vi "ConcatenateOntoShortcutMenu.vi"(8 "error in":errorcluster, 9 "menu ref in":refnum<k9>, 11 "Scope in":refnum<class "Scope Instrument.lvclass">) -> (0 "error out":errorcluster, 1 "menu ref out":refnum<k9>, 3 "Scope out":refnum<class "Scope Instrument.lvclass">)   [LabVIEW 2025, in "Scope.lvlib" / "Scope Instrument.lvclass"]
doc: "Allows children to insert menu items without overriding ShortcutMenu.vi entirely. By default, called after Add/Remove.Copyright 2017 National Instruments Corporation\n\nLicensed under the Apache License, Version 2.0 (the \"License\"); you may not use this file except in compliance with the License. You may obtain a copy of the License at http://www.apache.org/licenses/LICENSE-2.0\nUnless required by applicable law or agreed to in writing, software distributed under the License is distributed on an \"AS IS\" BASIS, WITHOUT WARRANTIES OR CONDITIONS OF ANY KIND, either express or implied. See the License for the specific language governing permissions and limitations under the License."
uses:
  Scope Instrument.lvclass
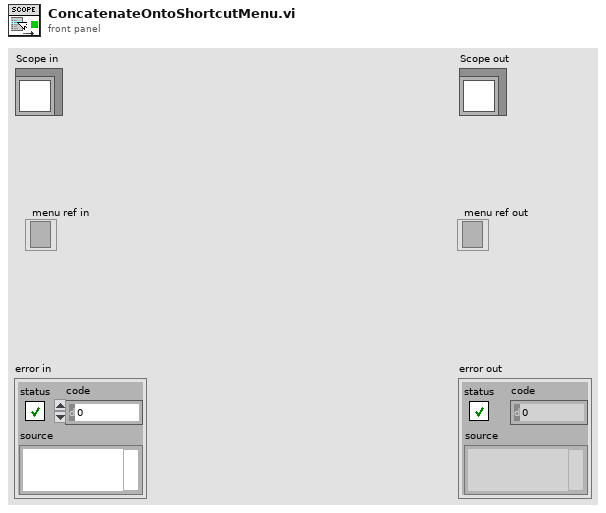
[diagram p1: front panel]
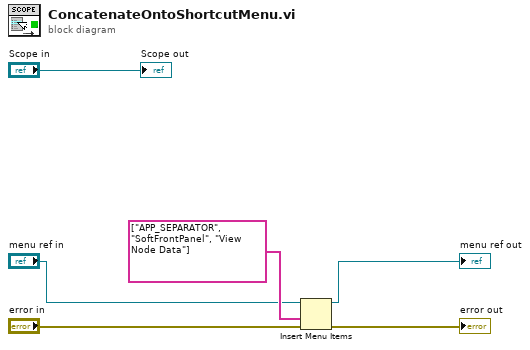
[diagram p0: block diagram]
diagram:
  n1 = Insert Menu Items(6:"error in", 7:string[] ["APP_SEPARATOR", "SoftFrontPanel", "View Node Data"], 9:"menu ref in") -> (0:→"error out":errorcluster, 3:→"menu ref out":refnum<k9>)  [unwired: 3 in, 1 out]
  "Scope out" <- "Scope in"
